vi "TAI_Solenoid.vi"(3 "Normal Output":bool, 4 "Override Actuator Bypass":bool, 5 "Actuator Name":string) -> (0 "Interlocked Output":bool, 2 "Output Mode":T1(ring))   [LabVIEW 2020]
doc: "This VI is configured for polymorphic use and functions as an interlock, allowing the selected solenoid to be tested manually via the FRC 4265 Dashboard. During testing, all interlocked actuators which are not selected for testing are disabled."
uses:
  driverdata.vi
  426a8fd3-0d55-4a18-942b-cc1f45a662fb.vi
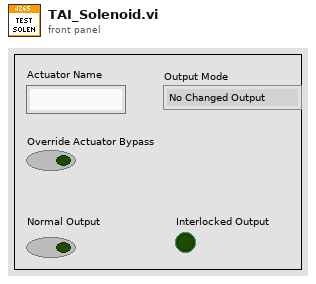
[diagram p1: front panel]
types:
  T1 = enum16{"No Changed Output", "New Normal Output", "New Testing Output"}
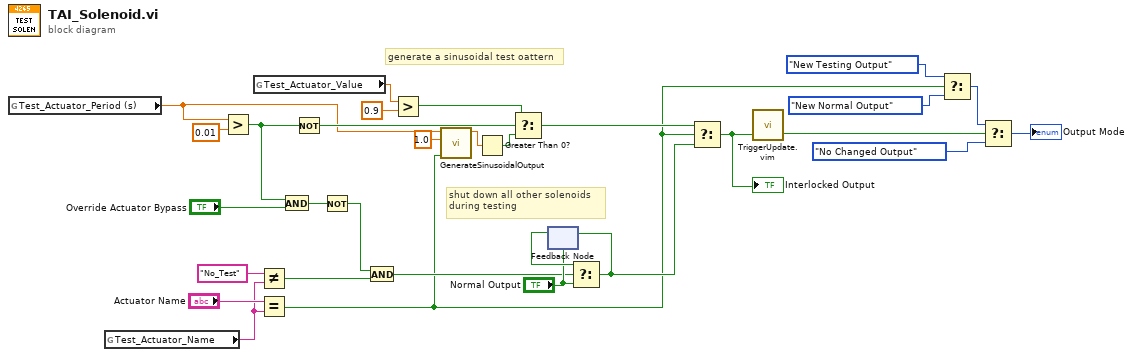
[diagram p0: block diagram]
diagram:
  # "generate a sinusoidal test oattern"
  # "shut down all other solenoids\nduring testing"
  n1 = global read "driverdata.vi" "Test_Actuator_Period (s)"() -> (w17:dbl)
  n2 = global read "driverdata.vi" "Test_Actuator_Name"() -> (w26:string)
  n3 = Greater?(x=w17, y=0.01) -> (0:w22:bool)
  n4 = global read "driverdata.vi" "Test_Actuator_Value"() -> (w18:dbl)
  n5 = Not Equal?(x="No_Test", y=w26) -> (x != y?=w10:bool)
  n6 = Equal?(x="Actuator Name", y=w26) -> (x = y?=w1:bool)
  n7 = And(x=w22, y="Override Actuator Bypass") -> (x .and. y?=w12:bool)
  n8 = Not(x=w22) -> (.not. x?=w21:bool)
  n9 = Not(x=w12) -> (.not. x?=w11:bool)
  n10 = And(x=w11, y=w10) -> (x .and. y?=w9:bool)
  n11 = Greater?(x=w18, y=0.9) -> (0:w19:bool)
  n12 = call "GenerateSinusoidalOutput.vi"("Init"=w1, "Amplitude"=1.0, "Period (s)"=w17) -> ("sin(time)"=w15:dbl)  [unwired: 8 in]
  n13 = Greater Than 0?(x=w15) -> (x > 0?=w14:bool)
  n14 = Select(t=w19, s=w21, f=w14) -> (s? t:f=w13:bool)
  n15 = feedback #1("Normal Output") -> (w27:bool)
  n16 = Select(t=w27, s=w9, f="Normal Output") -> (s? t:f=w28:bool)
  n17 = feedback-in #1(w28) -> ()
  n18 = Select(t=w13, s=w1, f=w28) -> (s? t:f=w2:bool)
  "Interlocked Output" <- w2
  n19 = call "TriggerUpdate.vim"("Trigger"=w2) -> ("Update"=w8:bool)  [unwired: 2 in]
  n20 = Select(t=T1."New Testing Output", s=w1, f=T1."New Normal Output") -> (s? t:f=w5:T1)
  n21 = Select(t=w5, s=w8, f=T1."No Changed Output") -> (s? t:f=→"Output Mode":T1)
